vi "About.vi"() -> ()   [LabVIEW 2013]
uses:
  Control/Buffer.vi
panel:
  out "Detail":string
  out "Version":string
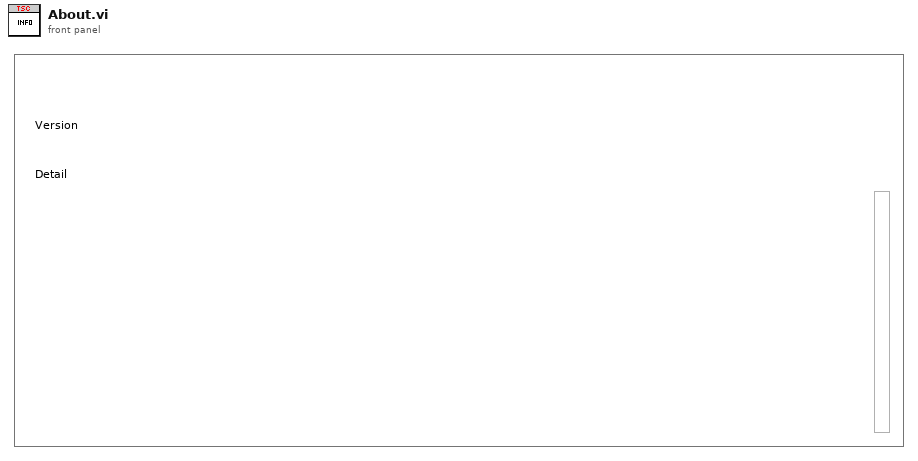
[diagram p1: front panel]
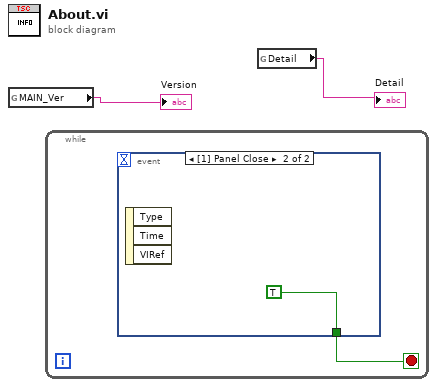
[diagram p0: block diagram]
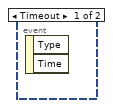
[diagram p2: hidden frame]
diagram:
  n1 = global read "Buffer.vi" "MAIN_Ver"() -> (→"Version":string)
  n2 = while {
    stop <- w3 stop-if-true
    n3 = event shown="[1] Panel Close" {
      selector: _ -> [_ _]
      dyn-events: _ -> [_ _]
      timeout: _ -> [_ _]
      tunnel: [_ TRUE] -> w3
      event Timeout {
        n4 = event-data() -> ()  [unwired: 3 out]
      }
      event Panel Close {
        n5 = event-data() -> ()  [unwired: 4 out]
      }
    }
  }
  n6 = global read "Buffer.vi" "Detail"() -> (→"Detail":string)
